vi "Close Hardware.vi"(8 "error in (no error)":errorcluster, 11 "Instrument.Oxford1820 in":refnum<class "Instrument.Oxford1820.lvclass">) -> (0 "error out":errorcluster, 3 "Instrument.Oxford1820 out":refnum<class "Instrument.Oxford1820.lvclass">)   [LabVIEW 2019, in "Instrument.Oxford1820.lvclass"]
uses:
  Instrument.Oxford1820.lvclass
  <instrlib>/Mercury iXX/Mercury iXX.lvlib
  <instrlib>/Mercury iXX/Public/Controls/Comms Transport Layer.ctl
  <instrlib>/Mercury iXX/Private/Controls/Query Dynamic Reference.ctl
  <instrlib>/Mercury iXX/Public/Controls/Mercury Reference.ctl
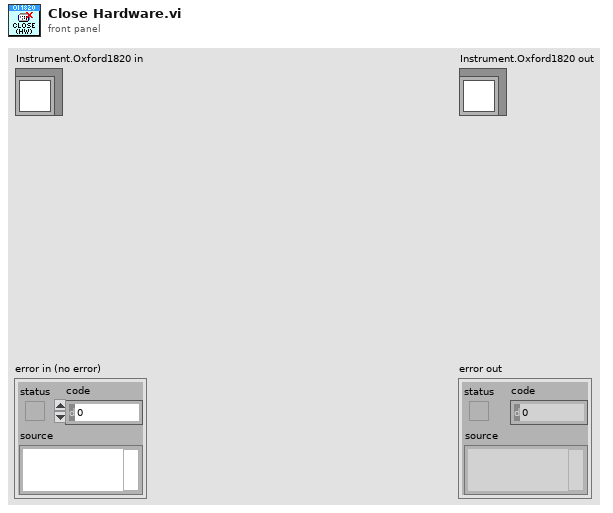
[diagram p1: front panel]
types:
  T1 = typedef "Mercury iXX.lvlib/Mercury Reference.ctl" = cluster{"Comms":refnum<visa-resource-name>, "Device ID":string[], "Comms Layer":T2, "Command":string, "Query reference":T3}
  T2 = typedef "Mercury iXX.lvlib/Comms Transport Layer.ctl" = enum16{"Ethernet TCP/IP", "USB", "ISOBus - RS-232", "GPIB"}
  T3 = typedef "Mercury iXX.lvlib/Query Dynamic Reference.ctl" = refnum<vi>
  T4 = cluster{"Address":string, "Reference":T1, "Devices":cluster{"Auxiliary":string, "Pressure":string, "Heater":string, "Temperature":string, "Lambda":string}}
  T5 = cluster{"Address":string, "Reference":T1, "Devices":cluster{"Level":string, "Temperature":string, "Magnet":string, "PSU1":string, "PSU 2":string, "PSU 3":string}}
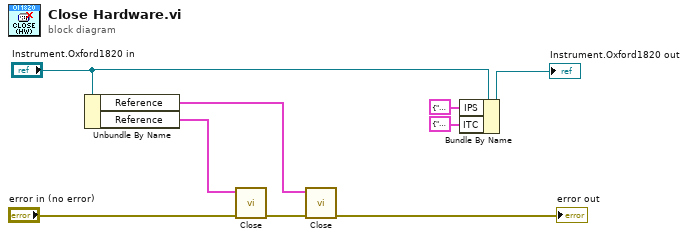
[diagram p0: block diagram]
diagram:
  n1 = Unbundle By Name("Instrument.Oxford1820 in") -> ("Reference"=w5:T1, "Reference"=w6:T1)
  n2 = call <instrlib>:"Close.vi"("error in (no error)"="error in (no error)", "Mercury Reference"=w6) -> ("error out"=w9:errorcluster)  [unwired: 9 out]
  n3 = call <instrlib>:"Close.vi"("error in (no error)"=w9, "Mercury Reference"=w5) -> ("error out"=→"error out":errorcluster)  [unwired: 9 out]
  n4 = Bundle By Name(cluster="Instrument.Oxford1820 in", "IPS"=T5 {"Address"="", "Reference"={"Comms"="", "Device ID"=[], "Comms Layer"=enum."Ethernet TCP/IP", "Command"="", "Query reference"=refnum}, "Devices"={"Level"="", "Temperature"="", "Magnet"="", "PSU1"="", "PSU 2"="", "PSU 3"=""}}, "ITC"=T4 {"Address"="", "Reference"={"Comms"="", "Device ID"=[], "Comms Layer"=enum."Ethernet TCP/IP", "Command"="", "Query reference"=refnum}, "Devices"={"Auxiliary"="", "Pressure"="", "Heater"="", "Temperature"="", "Lambda"=""}}) -> (→"Instrument.Oxford1820 out":refnum<class "Instrument.Oxford1820.lvclass">)
